vi "RunPedestalSubV1729A.vi"(4 "# Events to Avg":i32, 6 "# Samples after Trig":u16, 7 "Clock Divisor":u32=2, 8 "error in (no error)":errorcluster, 9 "handle in":i32, 10 "Init State":T1(ring), 11 "VME Base Address in":u32 format="%.0x") -> (0 "error out":errorcluster, 1 "handle out":i32, 2 "Data Out":u32[][](array[numeric]), 3 "Offset":i16)   [LabVIEW 2014]
uses:
  Program Files (x86)/CAEN/Comm/labview/CAENComm.lvlib
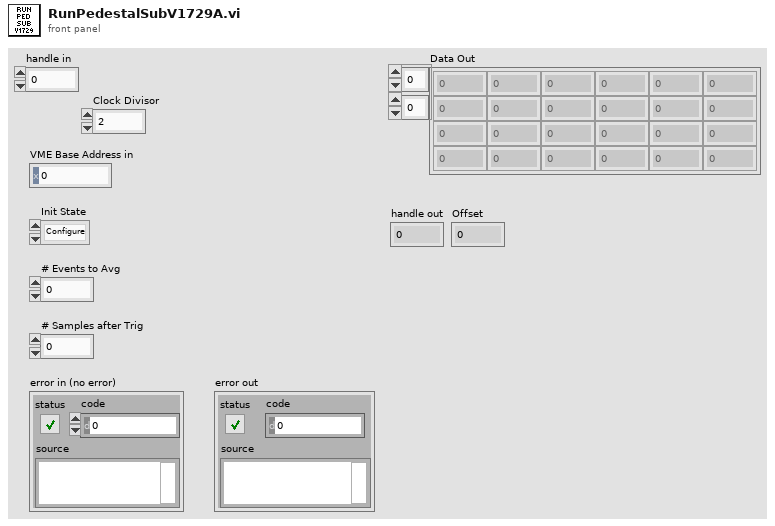
[diagram p1: front panel]
types:
  T1 = enum16{"Configure", "Initialise", "Run", "Close"}
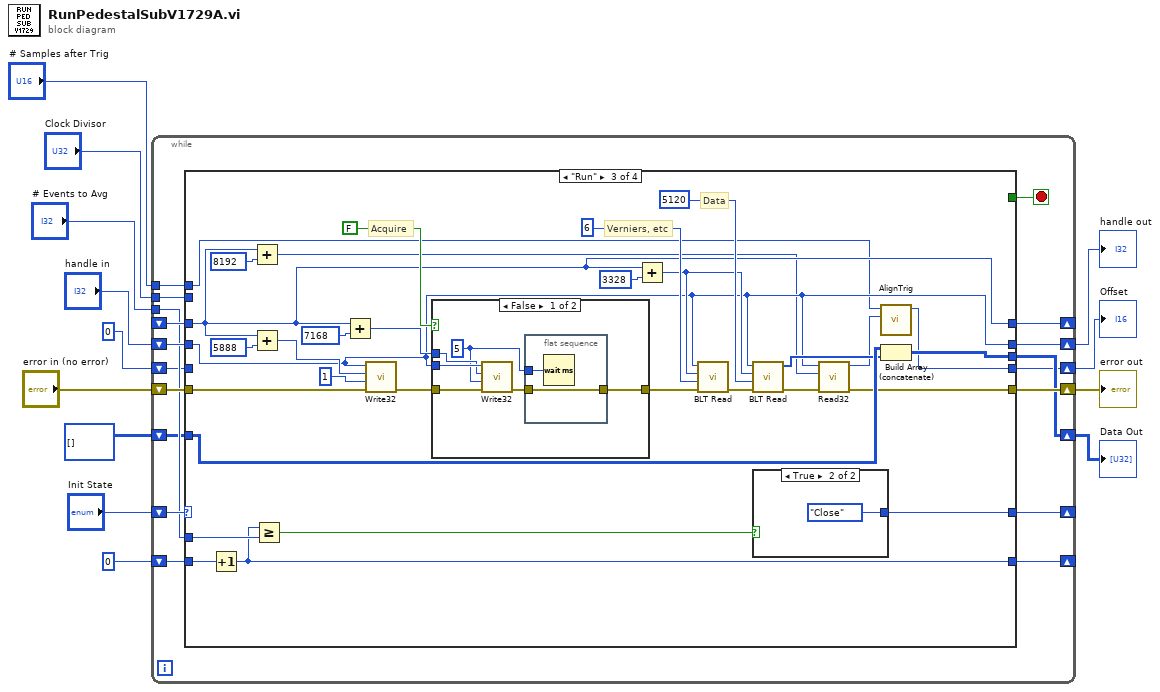
[diagram p0: block diagram]
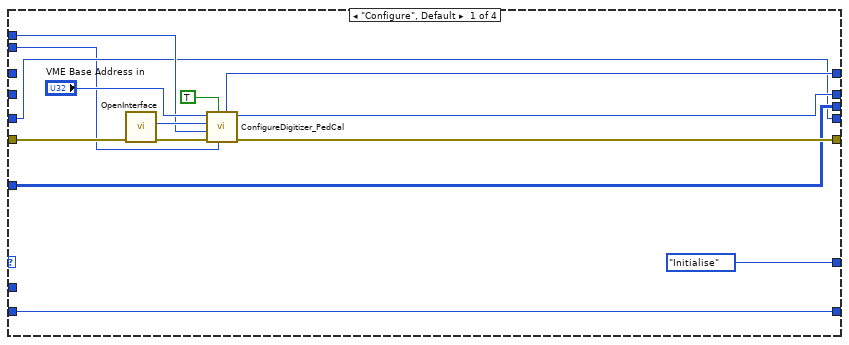
[diagram p2: hidden frame]
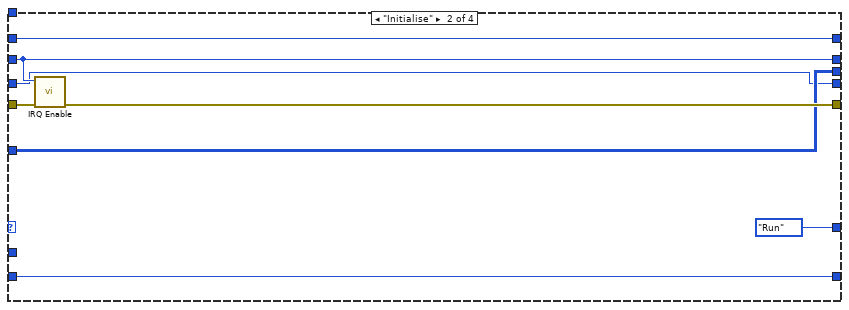
[diagram p3: hidden frame]
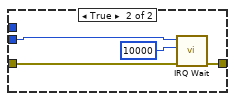
[diagram p4: hidden frame]
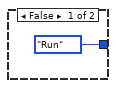
[diagram p5: hidden frame]
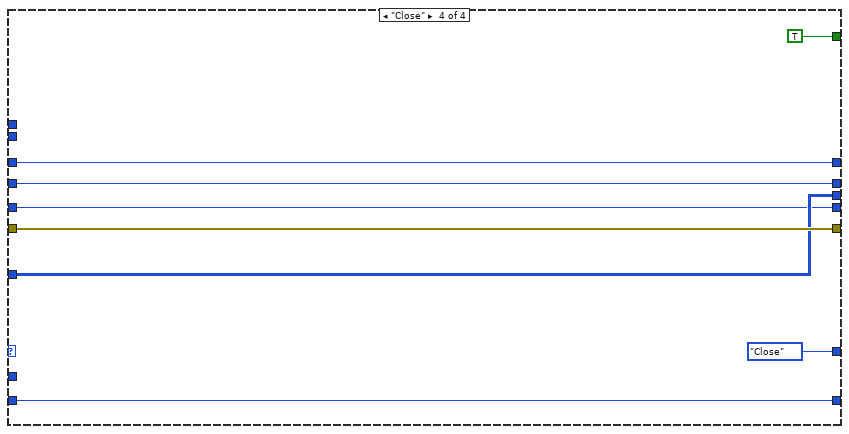
[diagram p6: hidden frame]
diagram:
  n1 = while {
    shift-right: [w24] -> _
    shift-left: "Init State" -> [w31]
    shift-right: [w29] -> w12
    shift-left: "error in (no error)" -> [w30]
    shift-right: [w28] -> _
    shift-left: _ -> [w25]
    shift-right: [w27] -> w4
    shift-left: "handle in" -> [w26]
    tunnel: "# Events to Avg" -> [w22]
    shift-right: [w20] -> _
    shift-left: 0 -> [w23]
    tunnel: "# Samples after Trig" -> [w19]
    shift-right: [w18] -> w6
    shift-left: u32[][] [] ("appended array") -> [w17]
    shift-right: [w16] -> w2
    shift-left: i16 0 ("Offset") -> [w15]
    tunnel: "Clock Divisor" -> [w14]
    stop <- w21 stop-if-true
    n2 = case shown="\"Run\"" w31 {
      tunnel: w30 -> [w45 w53 w80 w101]
      tunnel: [w42 w48 w61 w101] -> w29
      tunnel: [w39 w51 w58 w104] -> w28
      tunnel: [w38 w52 w60 w105] -> w27
      tunnel: w26 -> [_ w52 w60 w105]
      tunnel: w25 -> [_ w51 w58 w104]
      tunnel: [T1."Initialise" T1."Run" w78 T1."Close"] -> w24
      tunnel: w23 -> [w36 w49 w77 w102]
      tunnel: w22 -> [_ _ w76 _]
      tunnel: [_ _ _ TRUE] -> w21
      tunnel: [w36 w49 w75 w102] -> w20
      tunnel: w19 -> [w35 _ w55 _]
      tunnel: [w34 w47 w66 w100] -> w18
      tunnel: w17 -> [w34 w47 w68 w100]
      tunnel: [w33 w46 w54 w99] -> w16
      tunnel: w15 -> [w33 w46 _ w99]
      tunnel: w14 -> [w32 _ _ _]
      frame "Configure", Default {
        n3 = call "OpenInterface.vi"("error in (no error)"=w45) -> ("error out"=w44:errorcluster, "handle"=w43:i32)  [unwired: 8 in, 1 out]
        n4 = call "ConfigureDigitizer_PedCal.vi"("Clock Divisor"=w32, "Software Trig?"=TRUE, "error in (no error)"=w44, "# Samples after Trig"=w35, "handle"=w43, "VME Base Address"="VME Base Address in") -> ("error out"=w42:errorcluster, "handle out"=w38:i32, "VME Base Address out"=w39:u32)  [unwired: 3 in]
      }
      frame "Initialise" {
        n5 = call "IRQ Enable.vi"("error in (no error)"=w53, "handle"=w52) -> ("error out"=w48:errorcluster)  [unwired: 9 in]
      }
      frame "Run" {
        # "Data"
        # "Verniers, etc"
        # "Acquire"
        n6 = Increment(x=w77) -> (x+1=w75:i32)
        n7 = Add(x=w58, y=u32 8192 ("x")) -> (x+y=w57:u32)
        n8 = Add(x=w58, y=u32 5888 ("x")) -> (x+y=w82:u32)
        n9 = Greater Or Equal?(x=w75, y=w76) -> (x >= y?=w74:bool)
        n10 = Add(x=w58, y=u32 7168 ("x")) -> (x+y=w63:u32)
        n11 = call "Write32.vi"("error in (no error)"=w80, "Data"=u32 1, "Address"=w82, "handle"=w60) -> ("error out"=w84:errorcluster)  [unwired: 7 in]
        n12 = case shown="False" FALSE {
          tunnel: w84 -> [w88 w95]
          tunnel: [w85 w94] -> w73
          tunnel: w60 -> [w90 w93]
          tunnel: w63 -> [w89 _]
          frame False {
            w87 = u32 5 ("Data")
            n13 = call "Write32.vi"("error in (no error)"=w88, "Data"=w87, "Address"=w89, "handle"=w90) -> ("error out"=w86:errorcluster)  [unwired: 7 in]
            n14 = flat-sequence {
              tunnel: w87 -> [w91]
              tunnel: w86 -> [w92]
              tunnel: [w92] -> w85
              frame #0 {
                n15 = Wait (ms)(milliseconds to wait=w91) -> ()  [unwired: 1 out]
              }
            }
          }
          frame True {
            n16 = call "IRQ Wait.vi"("error in (no error)"=w95, "Timeout"=u32 10000, "handle"=w93) -> ("error out"=w94:errorcluster)  [unwired: 8 in]
          }
        }
        n17 = Add(x=w58, y=u32 3328 ("x")) -> (x+y=w69:u32)
        n18 = call "BLT Read.vi"("error in (no error)"=w73, "BltSize"=6, "Address"=w69, "handle"=w60) -> ("error out"=w72:errorcluster)  [unwired: 5 in, 2 out]
        n19 = call "BLT Read.vi"("error in (no error)"=w72, "BltSize"=5120, "Address"=w69, "handle"=w60) -> ("error out"=w62:errorcluster, "Buff"=w67:u32[])  [unwired: 5 in, 1 out]
        n20 = case shown="True" w74 {
          tunnel: [T1."Run" T1."Close"] -> w78
          frame False {
          }
          frame True {
          }
        }
        n21 = call "Read32.vi"("error in (no error)"=w62, "Address"=w57, "handle"=w60) -> ("error out"=w61:errorcluster, "Data"=w56:u32)  [unwired: 7 in]
        n22 = call "AlignTrig.vi"("TRIG_REC"=w56, "# Samples after Trig"=w55) -> ("Offset"=w54:i16)  [unwired: 9 in]
        n23 = Build Array (concatenate)(w68, w67) -> (w66:u32[][])
      }
      frame "Close" {
      }
    }
  }
  "error out" <- w12
  "Data Out" <- w6
  "handle out" <- w4
  "Offset" <- w2
